vi "WAM_RADIO_BUTTONS.vi"() -> (2 "Index out":u32)   [LabVIEW 2018]
panel:
  out "PanelClose?(t)":bool=TRUE
  in  "Radio Buttons":T1(radio)
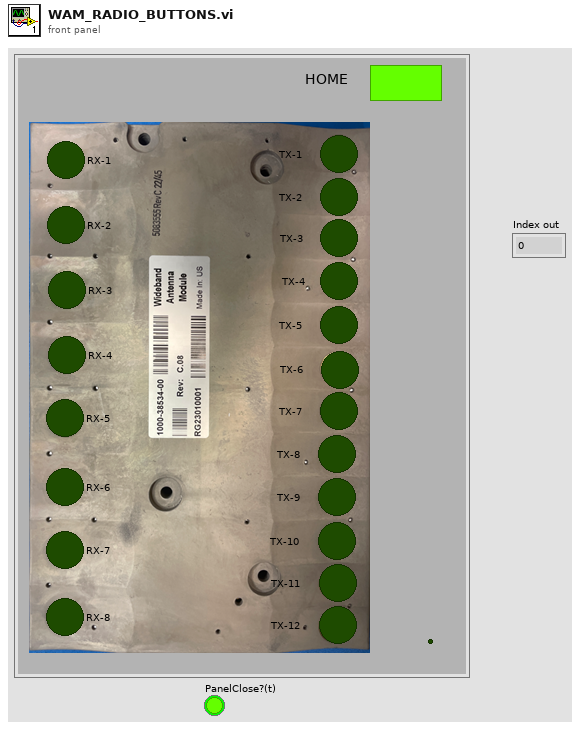
[diagram p1: front panel]
types:
  T1 = enum32{"HOME", "TX-1", "TX-2", "TX-3", "TX-4", "TX-5", "TX-6", "TX-7", "TX-8", "TX-9", "TX-10", "TX-11", "TX-12", "RX-8", "RX-7", "RX-6", "RX-5", "RX-4", "RX-3", "RX-2", "RX-1", "RX-8 2"}
  T2 = enum32{"Invalid", "Standard", "Closed", "Hidden", "Minimized", "Maximized"}
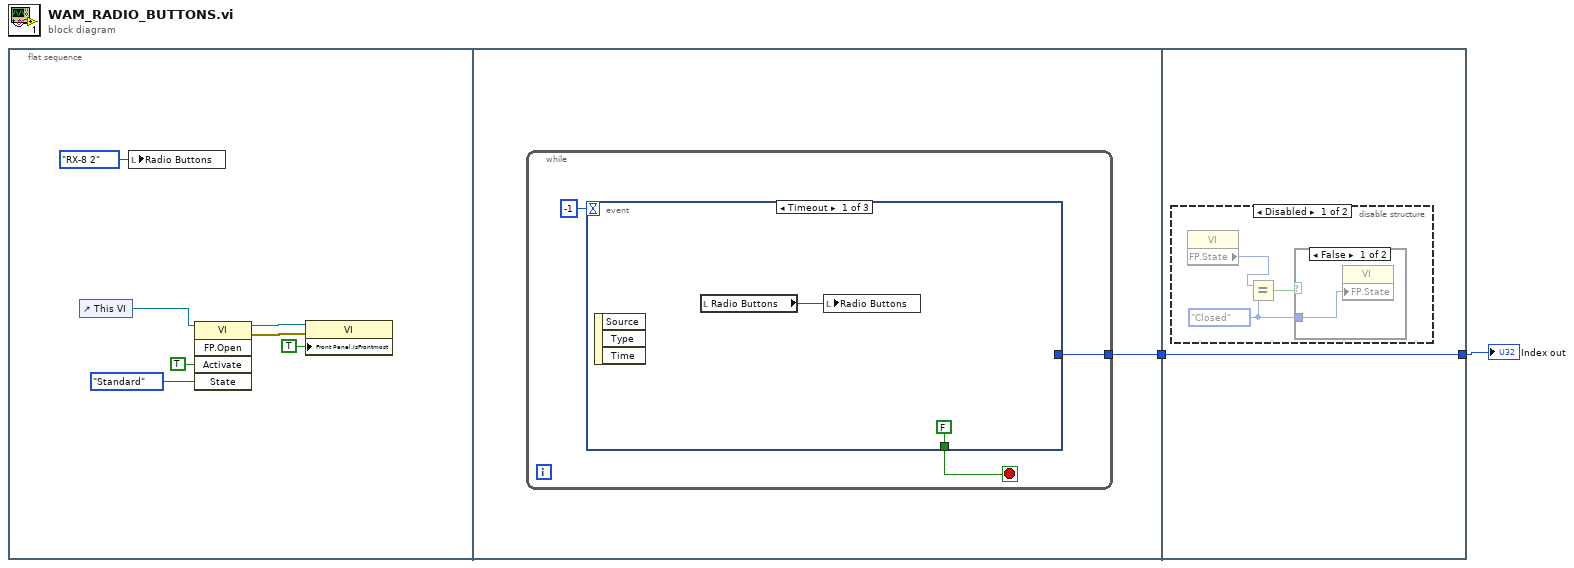
[diagram p0: block diagram]
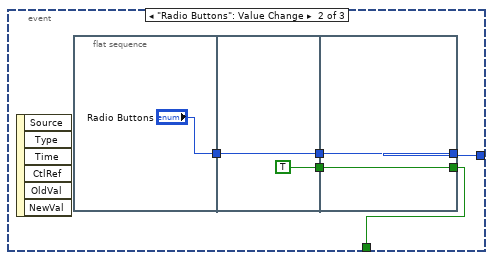
[diagram p2: hidden frame]
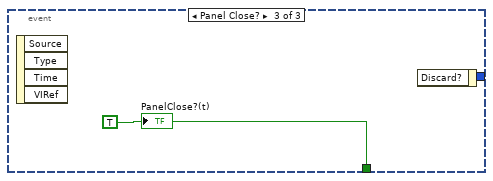
[diagram p3: hidden frame]
diagram:
  n1 = flat-sequence {
    tunnel: [w10] -> w2
    tunnel: [w27] -> w1
    tunnel: w2 -> [w27]
    frame #0 {
      n2 = control-ref of="This VI"() -> (w9:refnum<vi>)
      n3 = local write "Radio Buttons"(T1."RX-8 2" ("Radio Buttons")) -> ()
      n4 = invoke class="VI" method="FP.Open"(reference=w9, "Activate"=TRUE ("Activate?"), "State"=T2."Standard") -> (reference out=w6:refnum<vi>, error out=w5:errorcluster)  [unwired: 2 in, 3 out]
      n5 = property class="VI"(reference=w6, error in=w5, "Front Panel.IsFrontmost"=TRUE ("Front Panel Window:Is Frontmost")) -> ()  [unwired: 2 out]
    }
    frame #1 {
      n6 = while {
        tunnel: [w13] -> w10
        stop <- w12 stop-if-true
        n7 = event shown="[0] Timeout" {
          selector: _ -> [_ _ _]
          dyn-events: _ -> [_ _ _]
          timeout: -1 -> [_ _ _]
          tunnel: [_ w20 _] -> w13
          tunnel: [FALSE w18 w26] -> w12
          event Timeout {
            n8 = event-data() -> ()  [unwired: 1 in, 3 out]
            n9 = local read "Radio Buttons"() -> (w14:T1)
            n10 = local write "Radio Buttons"(w14) -> ()
          }
          event "Radio Buttons": Value Change {
            n11 = event-data() -> ()  [unwired: 1 in, 6 out]
            n12 = flat-sequence {
              tunnel: ["Radio Buttons"] -> w19
              tunnel: w19 -> [w23]
              tunnel: [w23] -> w17
              tunnel: [TRUE] -> w16
              tunnel: [w24] -> w18
              tunnel: [w25] -> w20
              tunnel: w17 -> [w25]
              tunnel: w16 -> [w24]
              frame #0 {
              }
              frame #1 {
              }
              frame #2 {
              }
            }
          }
          event Panel Close? {
            w26 = TRUE
            n13 = event-data() -> ()  [unwired: 1 in, 4 out]
            n14 = event-data() -> ()  [unwired: 2 in, 1 out]
            "PanelClose?(t)" <- w26
          }
        }
      }
    }
    frame #2 {
      n15 = disable-structure shown="Disabled" {
        frame Disabled {
          w30 = T2."Closed" ("Front Panel Window:State")
          n16 = property class="VI"() -> ("FP.State"=w29:T2)  [unwired: 2 in, 2 out]
          n17 = Equal?(x=w29, y=w30) -> (x = y?=w28:bool)
          n18 = case shown="False" w28 {
            tunnel: w30 -> [w31 _]
            frame False {
              n19 = property class="VI"("FP.State"=w31) -> ()  [unwired: 2 in, 2 out]
            }
            frame True {
            }
          }
        }
        frame Enabled {
        }
      }
    }
  }
  "Index out" <- w1
